vi "Library Absolve Resource Path.vi"(0 "alternate absolute base (none)":path, 7 "path in":path) -> (8 "absolved path":path)   [LabVIEW 2012]
doc: "Takes an input path and makes it absolute when it is relative or empty. When the path is already absolute, it is left unmodified. To make the path absolute, the configured resource base path is prepended. If the resource base path is empty or relative, the default absolute path is prepended to that (the source root in development mode, the application directory when built).\n\nResources are files or directories containing scripts, function VIs, plugin VIs or any other application data you might care to store under the same tree. This allows access to resource files without having to specify an absolute path everywhere, which is an utter pain when the resource directory must be migrated. For convenience, when no resource base path is specified or a relative base path is specified, the prepended path is the LuaVIEW directory in development mode and the application directory when deployed as a built application."
uses:
  glb_Library Configuration Globals.vi
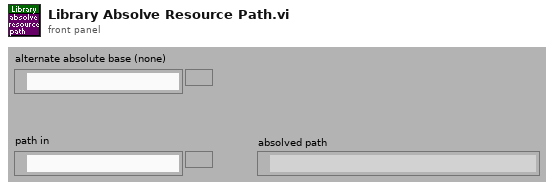
[diagram p1: front panel]
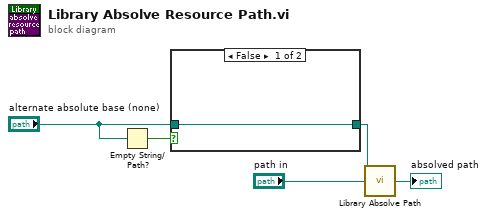
[diagram p0: block diagram]
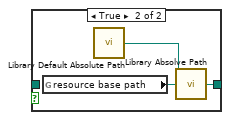
[diagram p2: hidden frame]
diagram:
  n1 = Empty String/Path?(string/path="alternate absolute base (none)") -> (empty?=w2:bool)
  n2 = case shown="False" w2 {
    tunnel: [w6 w7] -> w4
    tunnel: "alternate absolute base (none)" -> [w6 _]
    frame False {
    }
    frame True {
      n3 = global read "glb_Library Configuration Globals.vi" "resource base path"() -> (w8:path)
      n4 = call "Library Default Absolute Path.vi"() -> ("default absolute path"=w9:path)  [unwired: 15 in]
      n5 = call "Library Absolve Path.vi"("absolute base"=w9, "input path to absolve"=w8) -> ("absolved path"=w7:path)  [unwired: 13 in]
    }
  }
  n6 = call "Library Absolve Path.vi"("absolute base"=w4, "input path to absolve"="path in") -> ("absolved path"=→"absolved path":path)  [unwired: 13 in]
